vi "DashboardGetRobotMode.vi"(8 "Dashboard":refnum<k24>, 11 "error in":errorcluster) -> (0 "Response":cluster{"Message":string, "Succeed":bool}, 1 "Mode":i32(ring) items=["Disconnected"=0, "ConfirmSafety"=1, "Booting"=2, "PowerOff"=3, "PowerOn"=4, "Idle"=5, "BackDrive"=6, "Running"=7, "UpdatingFirmware"=8, "Other"=-1], 3 "error out":errorcluster)   [LabVIEW 2023, in "UnderAutomation.UniversalRobots.lvlib"]
uses:
  UnderAutomation.UniversalRobots.lvlib
  C:/Users/fg/Documents/UniversalRobots.vi/LabVIEW_2024/UnderAutomation.UniversalRobots/lib/UnderAutomation.UniversalRobots.dll
  LabVIEW_2024/UnderAutomation.UniversalRobots/lib/UnderAutomation.UniversalRobots.dll
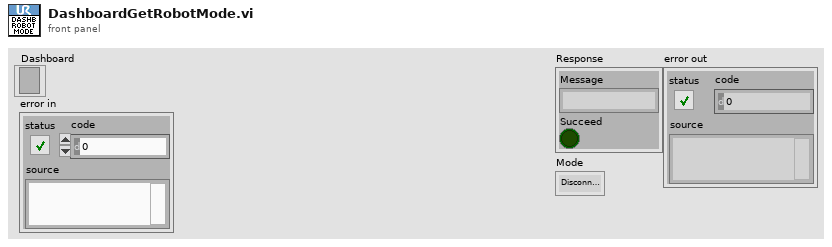
[diagram p1: front panel]
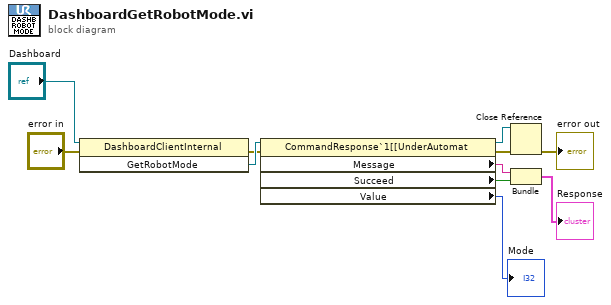
[diagram p0: block diagram]
diagram:
  n1 = invoke class="DashboardClientInternal" method="GetRobotMode"(reference="Dashboard", error in="error in") -> (error out=w7:errorcluster, "GetRobotMode"=w8:refnum<k24>)  [unwired: 1 in, 1 out]
  n2 = property class="CommandResponse`1[[UnderAutomat"(reference=w8, error in=w7) -> (reference out=w1:refnum<k24>, error out=w3:errorcluster, "Message"=w6:string, "Succeed"=w5:bool, "Value"=→"Mode":i32)
  n3 = Close Reference(reference=w1, error in (no error)=w3) -> (error out=→"error out":errorcluster)
  n4 = Bundle("Message"=w6, "Succeed"=w5) -> (→"Response":cluster{"Message":string, "Succeed":bool})  [unwired: 1 in]
